vi "GetDataForDataEvent.vi"(8 "error in (no error)":errorcluster, 10 "DataEvent":T4, 11 "service":refnum<class "IcmMessageService.lvclass">) -> (0 "error out":errorcluster, 2 "TrendPoints":T1[](array[typedef]), 3 "DataSets":T3[](array[typedef]))   [LabVIEW 2017]
uses:
  <vilib>/addons/InsightCM/MessageBus/MessageService/IcmMessageService.lvclass
  <vilib>/addons/InsightCM/MessageBus/Base/controls/DataEvent.ctl
  <vilib>/addons/InsightCM/MessageBus/Base/controls/KeyValuePair.ctl
  <vilib>/addons/InsightCM/MessageBus/Base/controls/DataSetByteData.ctl
  <vilib>/addons/InsightCM/MessageBus/Base/controls/TrendPoint.ctl
  <vilib>/addons/InsightCM/MessageBus/MessageLibrary/DataManagement/controls/DataManagementGetDataForDataEventRequestBody.ctl
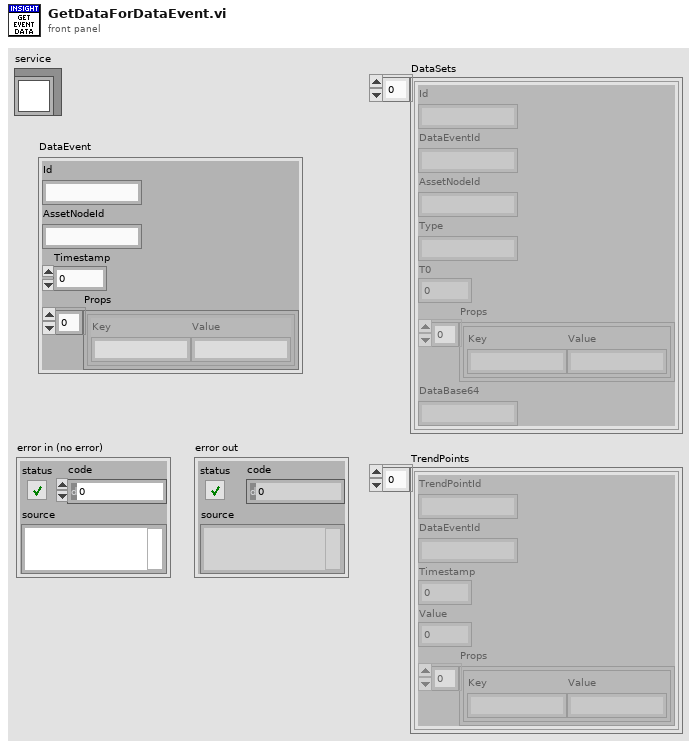
[diagram p1: front panel]
types:
  T1 = typedef "TrendPoint.ctl" = cluster{"TrendPointId":string, "DataEventId":string, "Timestamp":i64, "Value":dbl, "Props":T2[]}
  T2 = typedef "KeyValuePair.ctl" = cluster{"Key":string, "Value":string}
  T3 = typedef "DataSetByteData.ctl" = cluster{"Id":string, "DataEventId":string, "AssetNodeId":string, "Type":string, "T0":i64, "Props":T2[], "DataBase64":string}
  T4 = typedef "DataEvent.ctl" = cluster{"Id":string, "AssetNodeId":string, "Timestamp":i64, "Props":T2[]}
  T5 = typedef "DataManagementGetDataForDataEventRequestBody.ctl" = cluster{"DataEvent":T4}
  T6 = typedef "Message.ctl" = cluster{"Header":T7, "Body":u8[]}
  T7 = typedef "MessageHeader.ctl" = cluster{"MessageName":string, "Timestamp":i64, "CorrelationId":string, "ContentType":string, "RoutingKey":string, "Properties":T2[]}
  T8 = typedef "DataManagementGetDataForDataEventResponseBody.ctl" = cluster{"DataSets":T3[], "TrendPoints":T1[]}
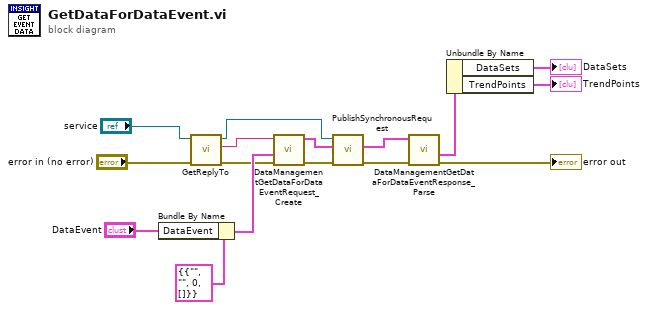
[diagram p0: block diagram]
diagram:
  n1 = Bundle By Name(cluster=T5 {"DataEvent"={"Id"="", "AssetNodeId"="", "Timestamp"=0, "Props"=[]}} ("DataManagementGetDataForDataEventRequest"), "DataEvent"="DataEvent") -> (w12:T5)
  n2 = call <vilib>:"GetReplyTo.vi"("error in (no error)"="error in (no error)", "service in"="service") -> ("error out"=w11:errorcluster, "reply to"=w9:string, "service out"=w16:refnum<class "IcmMessageService.lvclass">)  [unwired: 7 in]
  n3 = call <vilib>:"DataManagementGetDataForDataEventRequest_Create.vi"("error in (no error)"=w11, "DataManagementGetDataForDataEventRequest"=w12, "ReplyTo"=w9) -> ("error out"=w10:errorcluster, "Message"=w7:T6)  [unwired: 7 in]
  n4 = call <vilib>:"PublishSynchronousRequest.vi"("error in (no error)"=w10, "request"=w7, "service in"=w16) -> ("error out"=w6:errorcluster, "response"=w4:T6)  [unwired: 6 in, 1 out]
  n5 = call <vilib>:"DataManagementGetDataForDataEventResponse_Parse.vi"("error in (no error)"=w6, "Message"=w4) -> ("error out"=→"error out":errorcluster, "Body"=w3:T8)  [unwired: 6 in, 2 out]
  n6 = Unbundle By Name(w3) -> ("DataSets"=→"DataSets":T3[], "TrendPoints"=→"TrendPoints":T1[])
